vi "Read Param.vi"(8 "error in (no error)":errorcluster, 11 "MB_TCP in":refnum<class "Master CR.lvclass">) -> (0 "error out":errorcluster, 2 "Param":refnum<class "Param.lvclass">, 3 "MB_TCP out":refnum<class "Master CR.lvclass">)   [LabVIEW 2021, in "Master CR.lvclass"]
uses:
  Master CR.lvclass
  Master CR.lvclass/Master CR.ctl
  Param.lvclass
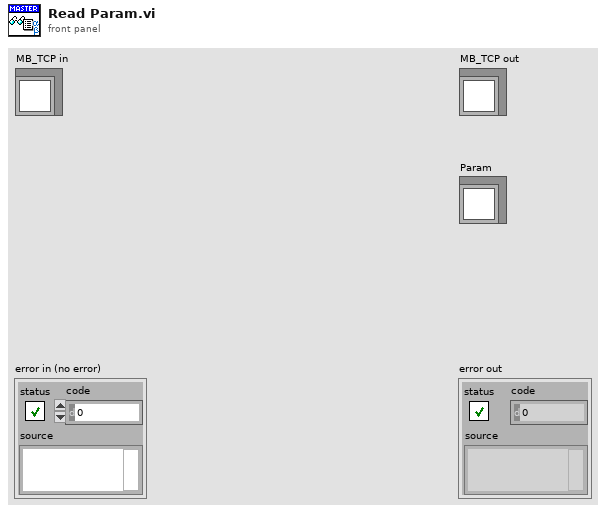
[diagram p1: front panel]
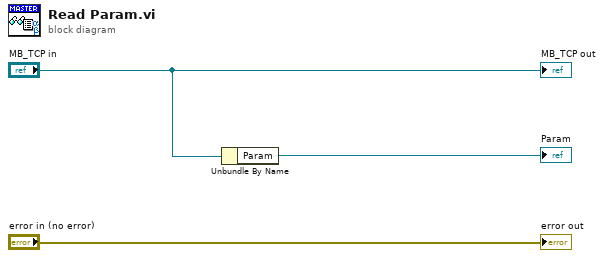
[diagram p0: block diagram]
diagram:
  n1 = Unbundle By Name("MB_TCP in") -> ("Param"=→"Param":refnum<class "Param.lvclass">)
  "error out" <- "error in (no error)"
  "MB_TCP out" <- "MB_TCP in"
